vi "pmu_Phasors Block.vi"(6 "init meas data":u8[](array[numeric]), 8 "measurement data":T1 {"trigger reason" format="%04b"}, 9 "data format":u16, 10 "phasor units":u32[](array[numeric]), 11 "nominal frequency":enum16{"50 Hz", "60 Hz"}(ring)) -> (0 "df/dt out of range":bool, 1 "freq out of range":bool, 2 "phasor out of range":bool, 3 "data block":u8[](array[numeric]) format="%b", 4 "analog out of range":bool)   [LabVIEW 2011, in "NI_EP_PMU.lvlib"]
doc: "This VI converts phasor data cluster to binary data block."
uses:
  <vilib>/addons/Electrical Power/PMU/NI_EP_PMU.lvlib
  <vilib>/addons/Electrical Power/PMU/Common/Controls/pmu_Measurement Data.ctl
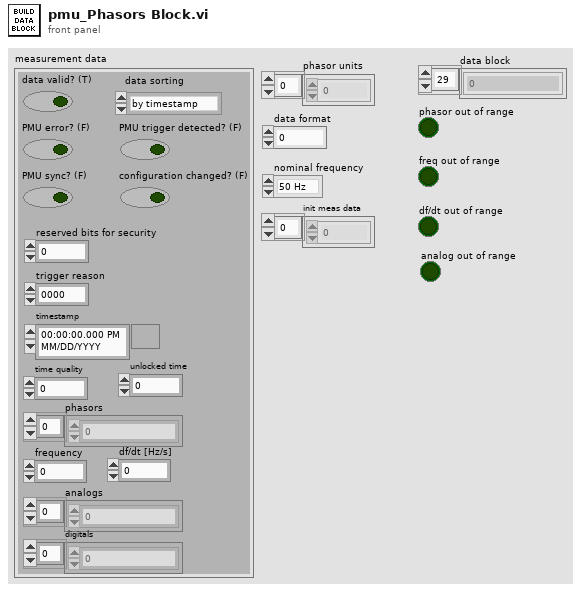
[diagram p1: front panel]
types:
  T1 = typedef "NI_EP_PMU.lvlib/pmu_Measurement Data.ctl" = cluster{"data valid? (T)":bool, "PMU error? (F)":bool, "PMU sync? (F)":bool, "data sorting":enum16{"by timestamp", "by arrival"}, "PMU trigger detected? (F)":bool, "configuration changed? (F)":bool, "df/dt [Hz/s]":sgl, "analogs":sgl[], "digitals":u16[], "frequency":sgl, "phasors":csg[], "reserved bits for security":u8, "trigger reason":u8, "timestamp":timestamp, "time quality":u8, "unlocked time":u32}
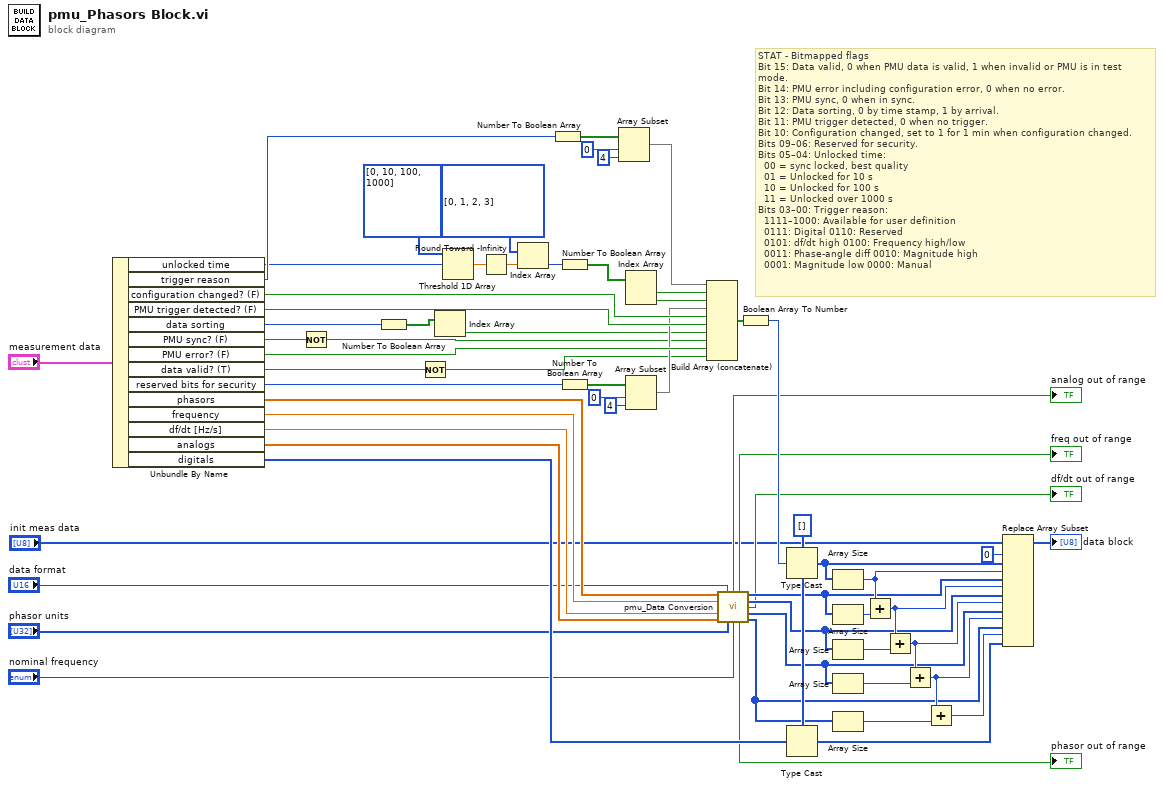
[diagram p0: block diagram]
diagram:
  w33 = u8[] [] ("appended array")
  # "STAT - Bitmapped flags\nBit 15: Data valid, 0 when PMU data is valid, 1 when invalid or PMU is in test mode.\nBit 14: PMU error including configuration error, 0 when no error.\nBit 13: PMU sync, 0 when in sync.\nBit 12: Data sorting, 0 by time stamp, 1 by arrival.\nBit 11: PMU trigger detected, 0 when no trigger.\nBit 10: Configuration changed, set to 1 for 1 min when configuration changed.\nBits 09–06: Reserved for security.\nBits 05–04: Unlocked time:\n  00 = sync locked, best quality\n  01 = Unlocked for 10 s\n  10 = Unlocked for 100 s\n  11 = Unlocked over 1000 s\nBits 03–00: Trigger reason:\n  1111–1000: Available for user definition\n  0111: Digital 0110: Reserved\n  0101: df/dt high 0100: Frequency high/low\n  0011: Phase-angle diff 0010: Magnitude high\n  0001: Magnitude low 0000: Manual"
  n1 = Unbundle By Name("measurement data") -> ("unlocked time"=w6:u32, "trigger reason"=w23:u8, "configuration changed? (F)"=w54:bool, "PMU trigger detected? (F)"=w53:bool, "data sorting"=w5:enum16{"by timestamp", "by arrival"}, "PMU sync? (F)"=w50:bool, "PMU error? (F)"=w51:bool, "data valid? (T)"=w52:bool, "reserved bits for security"=w49:u8, "phasors"=w21:csg[], "frequency"=w19:sgl, "df/dt [Hz/s]"=w17:sgl, "analogs"=w15:sgl[], "digitals"=w30:u16[])
  n2 = Not(x=w50) -> (.not. x?=w1:bool)
  n3 = Number To Boolean Array(number=w5) -> (Boolean array=w4:bool[])
  n4 = Not(x=w52) -> (.not. x?=w2:bool)
  n5 = Index Array(array=w4) -> (element=w3:bool)  [unwired: 1 in]
  n6 = Threshold 1D Array(2:w6, 3:u32[] [0, 10, 100, 1000]) -> (0:w62:dbl)  [unwired: 1 in]
  n7 = Round Toward -Infinity(1:w62) -> (0:w61:dbl)
  n8 = Index Array(array=u8[] [0, 1, 2, 3], index=w61) -> (element=w58:u8)
  n9 = Number To Boolean Array(number=w23) -> (Boolean array=w26:bool[])
  n10 = Number To Boolean Array(number=w58) -> (Boolean array=w57:bool[])
  n11 = Number To Boolean Array(number=w49) -> (Boolean array=w48:bool[])
  n12 = Array Subset(array=w26, index=0, length=4) -> (w25:bool[])
  n13 = Index Array(array=w57) -> (element #1=w56:bool, element #2=w55:bool)  [unwired: 2 in]
  n14 = Array Subset(array=w48, index=0, length=4) -> (w45:bool[])
  n15 = Build Array (concatenate)(w25, w56, w55, w45, w54, w53, w3, w1, w51, w2) -> (w63:bool[])
  n16 = call <vilib>:"pmu_Data Conversion.vi"("phasors in"=w21, "format"="data format", "freq in"=w19, "dfreq in"=w17, "analogs in"=w15, "phasor units"="phasor units", "nominal frequency"="nominal frequency") -> ("analog out of range"=→"analog out of range":bool, "freq out of range"=→"freq out of range":bool, "phasor byte array"=w20:u8[], "freq byte array"=w18:u8[], "df/dt out of range"=→"df/dt out of range":bool, "dfreq byte array"=w16:u8[], "phasor out of range"=→"phasor out of range":bool, "analogs byte array"=w14:u8[])  [unwired: 1 in]
  n17 = Boolean Array To Number(Boolean array=w63) -> (number=w31:u16)
  n18 = Type Cast(type=w33, x=w31) -> (*(type *) &x=w43:u8[])
  n19 = Type Cast(type=w33, x=w30) -> (*(type *) &x=w32:u8[])
  n20 = Array Size(array=w43) -> (size(s)=w41:i32)
  n21 = Array Size(array=w20) -> (size(s)=w42:i32)
  n22 = Array Size(array=w18) -> (size(s)=w40:i32)
  n23 = Array Size(array=w16) -> (size(s)=w38:i32)
  n24 = Array Size(array=w14) -> (size(s)=w36:i32)
  n25 = Add(x=w41, y=w42) -> (x+y=w39:i32)
  n26 = Add(x=w39, y=w40) -> (x+y=w37:i32)
  n27 = Add(x=w37, y=w38) -> (x+y=w35:i32)
  n28 = Add(x=w35, y=w36) -> (x+y=w34:i32)
  n29 = Replace Array Subset(array="init meas data", new element #1=w43, index #1=0 ("index"), new element #2=w20, index #2=w41, new element #3=w18, index #3=w39, new element #4=w16, index #4=w37, new element #5=w14, index #5=w35, new element #6=w32, index #6=w34) -> (→"data block":u8[])
